vi "AutoSetLEDemands.vi"(8 "error in (no error)":errorcluster, 9 "SetExtendPositonDemand(in)":dbl, 10 "SetLIftPostionDemand(d)":dbl) -> (0 "error out":errorcluster)   [LabVIEW 2020]
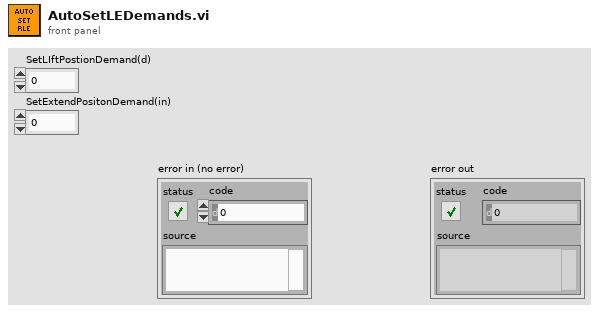
[diagram p1: front panel]
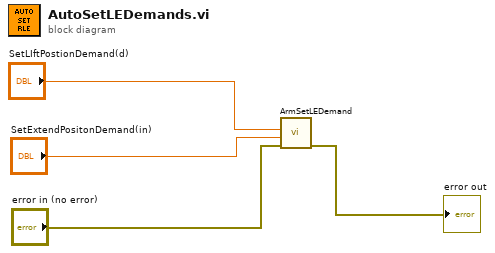
[diagram p0: block diagram]
diagram:
  n1 = call "ArmSetLEDemand.vi"("error in (no error)"="error in (no error)", "SetExtendPositonDemand(in)"="SetExtendPositonDemand(in)", "SetLIftPostionDemand(d)"="SetLIftPostionDemand(d)") -> ("error out"=→"error out":errorcluster)  [unwired: 8 in]
